vi "LVClass_CorrectionDataManager GetDeltaCommandsFromDeltaSlopes.vi"(0 "CorrectionDataManager in":refnum<class "CorrectionDataManager.lvclass">, 5 "Delta Slopes IN":refnum<class "HasoSlopes.lvclass">, 11 "error in (no error)":errorcluster) -> (4 "CorrectionDataManager out":refnum<class "CorrectionDataManager.lvclass">, 6 "Delta Slope OUT":refnum<class "HasoSlopes.lvclass">, 10 "DeltaPosition":T1, 15 "error out":errorcluster)   [LabVIEW 2020, in "CorrectionDataManager.lvclass"]
doc: "Compute the relative wavefront corrector commands corresponding to a\ndelta_slopes variation.\n\n<B>corrdata_managerIn</B> : CorrDataManager object.\n<B>corrdata_managerOut</B> : CorrDataManager object.\n<B>delta_slopes</B> : Slopes delta (stored as HasoSlopes).\n<B>delta_command</B> : Array of size actuators count, containing the commands deltas (relatives\n variations to apply from actuators initial positions)."
uses:
  CorrectionDataManager.lvclass
  HasoSlopes/HasoSlopes.lvclass
  Controls/Wavefront Corrector Position.ctl
  CorrectionDataManager.lvclass/CorrectionDataManager.ctl
  HasoSlopes/LVClass_HasoSlopes Read HasoSlopes _ property.vi
panel:
  # "WavefrontCorrectorOffsetState not be used"
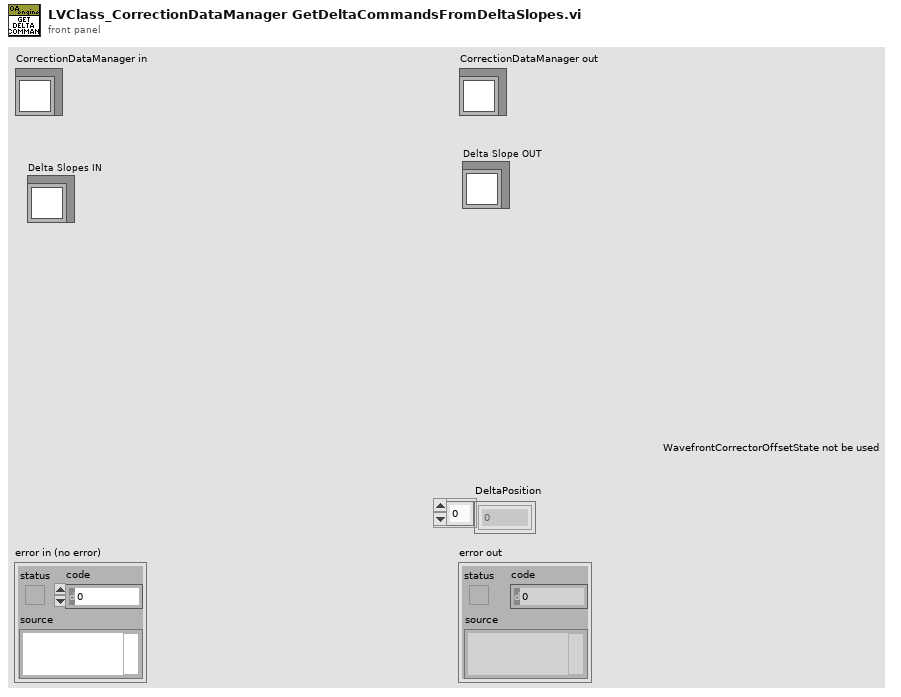
[diagram p1: front panel]
types:
  T1 = typedef "Wavefront Corrector Position.ctl" = sgl[]
  T2 = typedef "ClassID.ctl" = i64
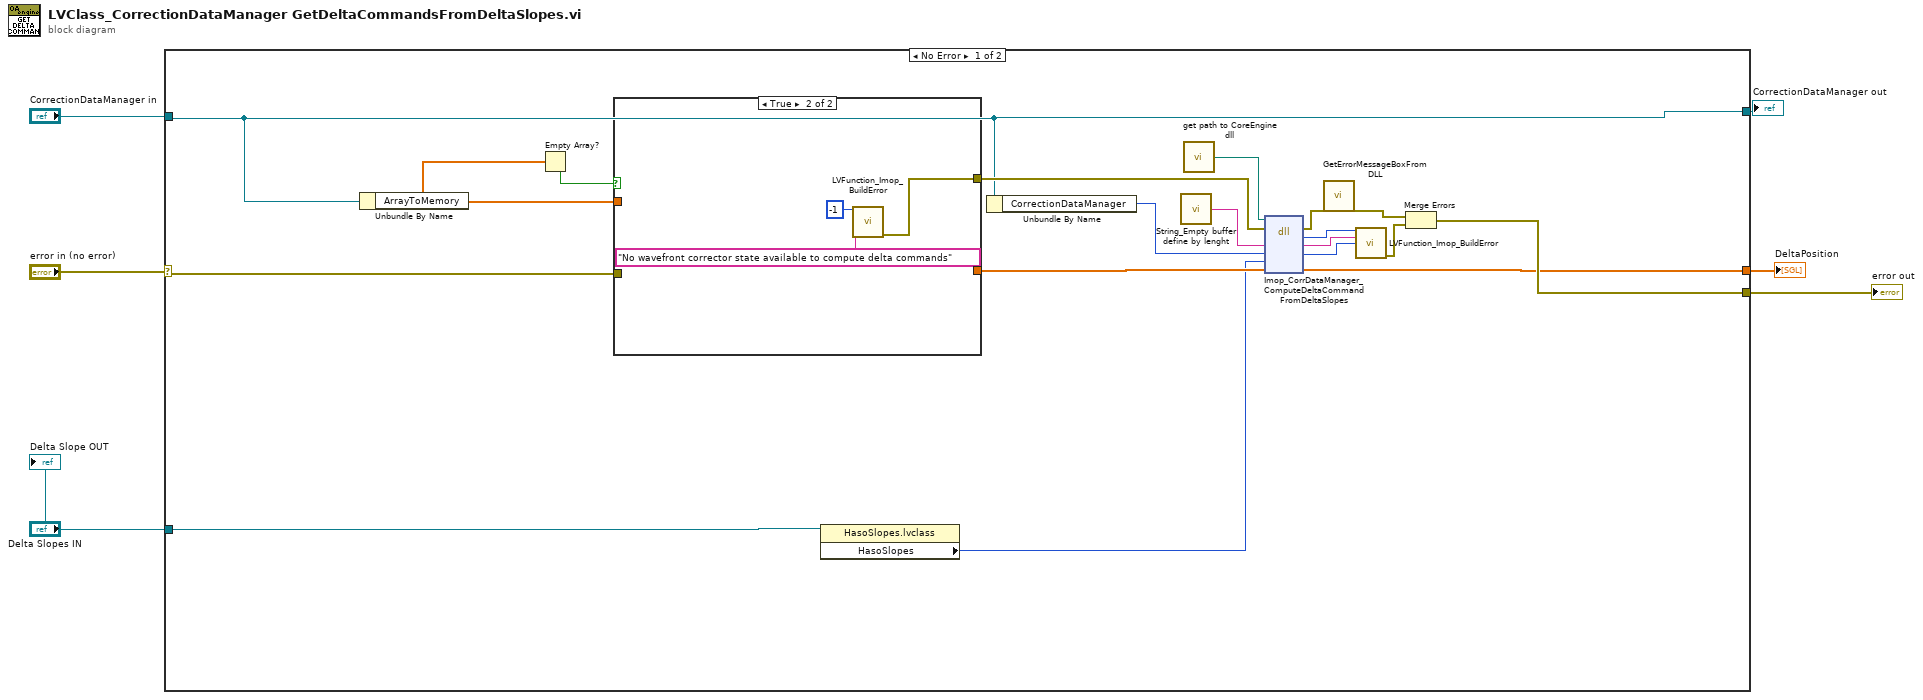
[diagram p0: block diagram]
diagram:
  n1 = case shown="No Error" "error in (no error)" {
    selector: "error in (no error)" -> [w17 w32]
    tunnel: [w18 w32] -> w6
    tunnel: [w8 w31] -> w5
    tunnel: "CorrectionDataManager in" -> [w8 w31]
    tunnel: "Delta Slopes IN" -> [w11 _]
    tunnel: [w12 _] -> w1
    frame No Error {
      n2 = Unbundle By Name(w8) -> ("ArrayToMemory"=w13:T1)
      n3 = Empty Array?(array=w13) -> (empty?=w9:bool)
      n4 = case shown="True" w9 {
        tunnel: w17 -> [w26 _]
        tunnel: [w26 w30] -> w16
        tunnel: [w27 _] -> w14
        tunnel: w13 -> [w27 _]
        frame False {
        }
        frame True {
          n5 = call "LVFunction_Imop_BuildError.vi"("code"=-1, "String to Prepend to source (\"\")"="No wavefront corrector state available to compute delta commands" ("String to Prepend to source (\"\")")) -> ("error out"=w30:errorcluster)  [unwired: 13 in]
        }
      }
      n6 = property class="HasoSlopes.lvclass"(reference=w11) -> ("HasoSlopes"=w10:T2)  [unwired: 1 in, 2 out]
      n7 = Unbundle By Name(w8) -> ("CorrectionDataManager"=w15:T2)
      n8 = call "String_Empty buffer define by lenght.vi"() -> ("Empty buffer"=w23:string)  [unwired: 1 in]
      n9 = call "get path to CoreEngine dll.vi"() -> ("path to wavekit library"=w22:path)  [unwired: 14 in, 1 out]
      n10 = dll-call lib="D:/FLE/0.Code/CoreEngine4_Suite/LV2011_interface/DLLs/c_interface_vc100.dll" fn="Imop_CorrDataManager_ComputeDeltaCommandFromDeltaSlopes"(path in=w22, error in=w16, "message"=w23, "WavefrontCorrection"=w15, "DeltaHasoSlopes"=w10, "delta_commands"=w14) -> (error out=w21:errorcluster, "return type"=w25:i32, "message"=w24:string, "WavefrontCorrection"=w7:i64, "delta_commands"=w12:sgl[])  [unwired: 2 in, 1 out]
      n11 = call "GetErrorMessageBoxFromDLL.vi"("error IN"=w21) -> ("error OUT"=w20:errorcluster)  [unwired: 10 in]
      n12 = call "LVFunction_Imop_BuildError.vi"("code"=w25, "String to Prepend to source (\"\")"=w24, "Adresse"=w7) -> ("error out"=w19:errorcluster)  [unwired: 12 in]
      n13 = Merge Errors(w20, w19) -> (w18:errorcluster)
    }
    frame Error {
    }
  }
  "error out" <- w6
  "CorrectionDataManager out" <- w5
  "DeltaPosition" <- w1
  "Delta Slope OUT" <- "Delta Slopes IN"
